vi "Get Error.vi"(11 "Hello World Queue in":refnum<class "Hello World Queue.lvclass">) -> (2 "Error":errorcluster)   [LabVIEW 2021, in "Hello World Queue.lvlib" / "Hello World Queue.lvclass"]
uses:
  Hello World Queue.lvclass
  Hello World Queue.lvclass/Hello World Queue.ctl
  jettl/Queue/Queue.lvclass
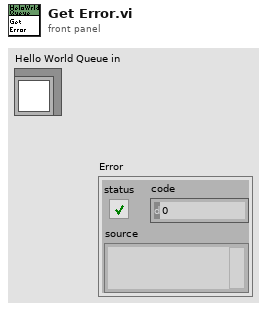
[diagram p1: front panel]
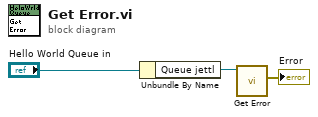
[diagram p0: block diagram]
diagram:
  n1 = Unbundle By Name("Hello World Queue in") -> ("Queue jettl"=w2:refnum<class "Queue.lvclass">)
  n2 = call-dynamic "Get Error.vi"("jettl in"=w2) -> ("Error"=→"Error":errorcluster)  [unwired: 10 in]
